vi "PPAS_DRIVE_EXECUTE.vi"(6 "Pass_Through_Time":dbl=-1.0 format="%33.4f", 8 "error in (no error)":errorcluster) -> (0 "error out":errorcluster)   [LabVIEW 2019]
uses:
  <vilib>/Rock Robotics/WPI/ThirdParty/JAS_Junk/TrajLib/Trajectory_Library.lvlib
  PPAS_DRIVE_GLOBALS.vi
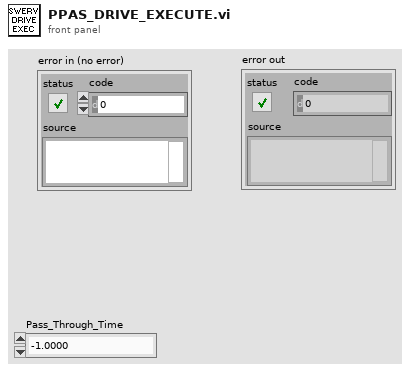
[diagram p1: front panel]
types:
  T1 = typedef "PPAS_DRIVE_MODULE_TYPDEF.ctl" = cluster{"SwervDriveMotor":T2, "SwerveSwerveMotor":T2, "SwerveDriveEnc":T7, "SwerveSwerveEnc":T7}
  T2 = typedef "WPI_MotorControlDeviceRef.ctl" = cluster{"DeviceStatus":errorcluster, "Type":T3, "PWM":cluster{"PWM Channel":T4, "DeadBand":T5}, "CAN":cluster{"Device Number":u8, "SetOutput VI Ref":variant, "GetOutput VI Ref":variant, "Enable VI Ref":variant, "Disable VI Ref":variant, "Data":variant}, "Invert":bool, "DIO PWM":cluster{"PWM \"Enable\" Channel":T4, "DIOChannel":T6, "PWM Rate":dbl}}
  T3 = typedef "WPI_MotorControlType.ctl" = enum16{"PWM", "CAN", "DIO PWM"}
  T4 = typedef "FPGA_DIOPWMChannel.ctl" = enum8{"PWM 0", "PWM 1", "PWM 2", "PWM 3", "PWM 4", "PWM 5", "PWM 6", "PWM 7", "PWM 8", "PWM 9", "PWM MXP 0", "PWM MXP 1", "PWM MXP 2", "PWM MXP 3", "PWM MXP 4", "PWM MXP 5", "PWM MXP 6", "PWM MXP 7", "PWM MXP 8", "PWM MXP 9", "Invalid"}
  T5 = typedef "WPI_PWMDeadband.ctl" = cluster{"Name":string, "maxPositivePwm":i32, "minPositivePwm":i32, "centerPwm":i32, "maxNegativePwm":i32, "minNegativePwm":i32, "angularRange":u16}
  T6 = typedef "FPGA_DIOChannel.ctl" = enum8{"DIO 0", "DIO 1", "DIO 2", "DIO 3", "DIO 4", "DIO 5", "DIO 6", "DIO 7", "DIO 8", "DIO 9", "DIO MXP 0", "DIO MXP 1", "DIO MXP 2", "DIO MXP 3", "DIO MXP 4", "DIO MXP 5", "DIO MXP 6", "DIO MXP 7", "DIO MXP 8", "DIO MXP 9", "DIO MXP 10", "DIO MXP 11", "DIO MXP 12", "DIO MXP 13", "DIO MXP 14", "DIO MXP 15", "SPI Port CS1", "SPI Port CS2", "SPI Port CS3", "SPI Port MISO", "SPI Port MOSI", "Invalid"}
  T7 = typedef "WPI_EncoderDevRef.ctl" = cluster{"DevStatus":errorcluster, "EncoderIndex":T8, "CounterIndex":T9, "DistancePerCount":dbl, "Decoding Type":T10}
  T8 = typedef "FPGA_EncoderIdx.ctl" = enum8{"Enc 0", "Enc 1", "Enc 2", "Enc 3", "Enc 4", "Enc 5", "Enc 6", "Enc 7", "Invalid"}
  T9 = typedef "FPGA_CounterCtrSystemIndex.ctl" = enum8{"Ctr 0", "Ctr 1", "Ctr 2", "Ctr 3", "Ctr 4", "Ctr 5", "Ctr 6", "Ctr 7", "Invalid"}
  T10 = typedef "WPI_EncoderType.ctl" = enum16{"1x", "2x", "4x"}
  T11 = typedef "WPI_GyroDevRef.ctl" = cluster{"DevStatus":errorcluster, "Analog Channel":T12, "Gain (VoltsPerDegree/Second)":dbl, "Gyro Type":enum16{"Analog", "XRS450"}, "Handle":i32, "SPI Bus":T13, "Device Found":bool, "Sample Rate":dbl, "Calibrate On Open":bool, "Offset":dbl}
  T12 = typedef "FPGA_AIChannel.ctl" = enum8{"AI 0", "AI 1", "AI 2", "AI 3", "AI MXP 0", "AI MXP 1", "AI MXP 2", "AI MXP 3", "Invalid"}
  T13 = typedef "spi_bus.ctl" = enum16{"SPI On-Board, CS0", "SPI On-Board, CS1", "SPI On-Board, CS2", "SPI On-Board, CS3", "SPI MXP", "Invalid"}
  T14 = typedef "Trajectory_Library.lvlib/SWERVE_DRIVE_MODULE_STATE.ctl" = cluster{"Speed":dbl, "Angle":T15}
  T15 = typedef "Trajectory_Library.lvlib/ROTATION2D.ctl" = cluster{"VALUE":dbl, "COS":dbl, "SIN":dbl}
  T16 = typedef "Trajectory_Library.lvlib/SWERVE_DRIVE_MODULE_POSITION.ctl" = cluster{"Distance":dbl, "Angle":T15, "P":bool}
  T17 = typedef "Trajectory_Library.lvlib/SWERVE_DRIVE_KINEMATICS.ctl" = cluster{"NumModules":i32, "InverseKinematics":T18, "ForwardKinematics":T18, "Modules":T19[], "PrevCoR":T19, "SavedModuleStates":T14[]}
  T18 = typedef "NI_Matrix.lvlib/RealMatrix.ctl" = dbl[][]
  T19 = typedef "Trajectory_Library.lvlib/TRANSLATION2D.ctl" = cluster{"X":dbl, "Y":dbl}
  T20 = typedef "Trajectory_Library.lvlib/CHASSIS_SPEEDS.ctl" = cluster{"vX":dbl, "vY":dbl, "vOmega":dbl}
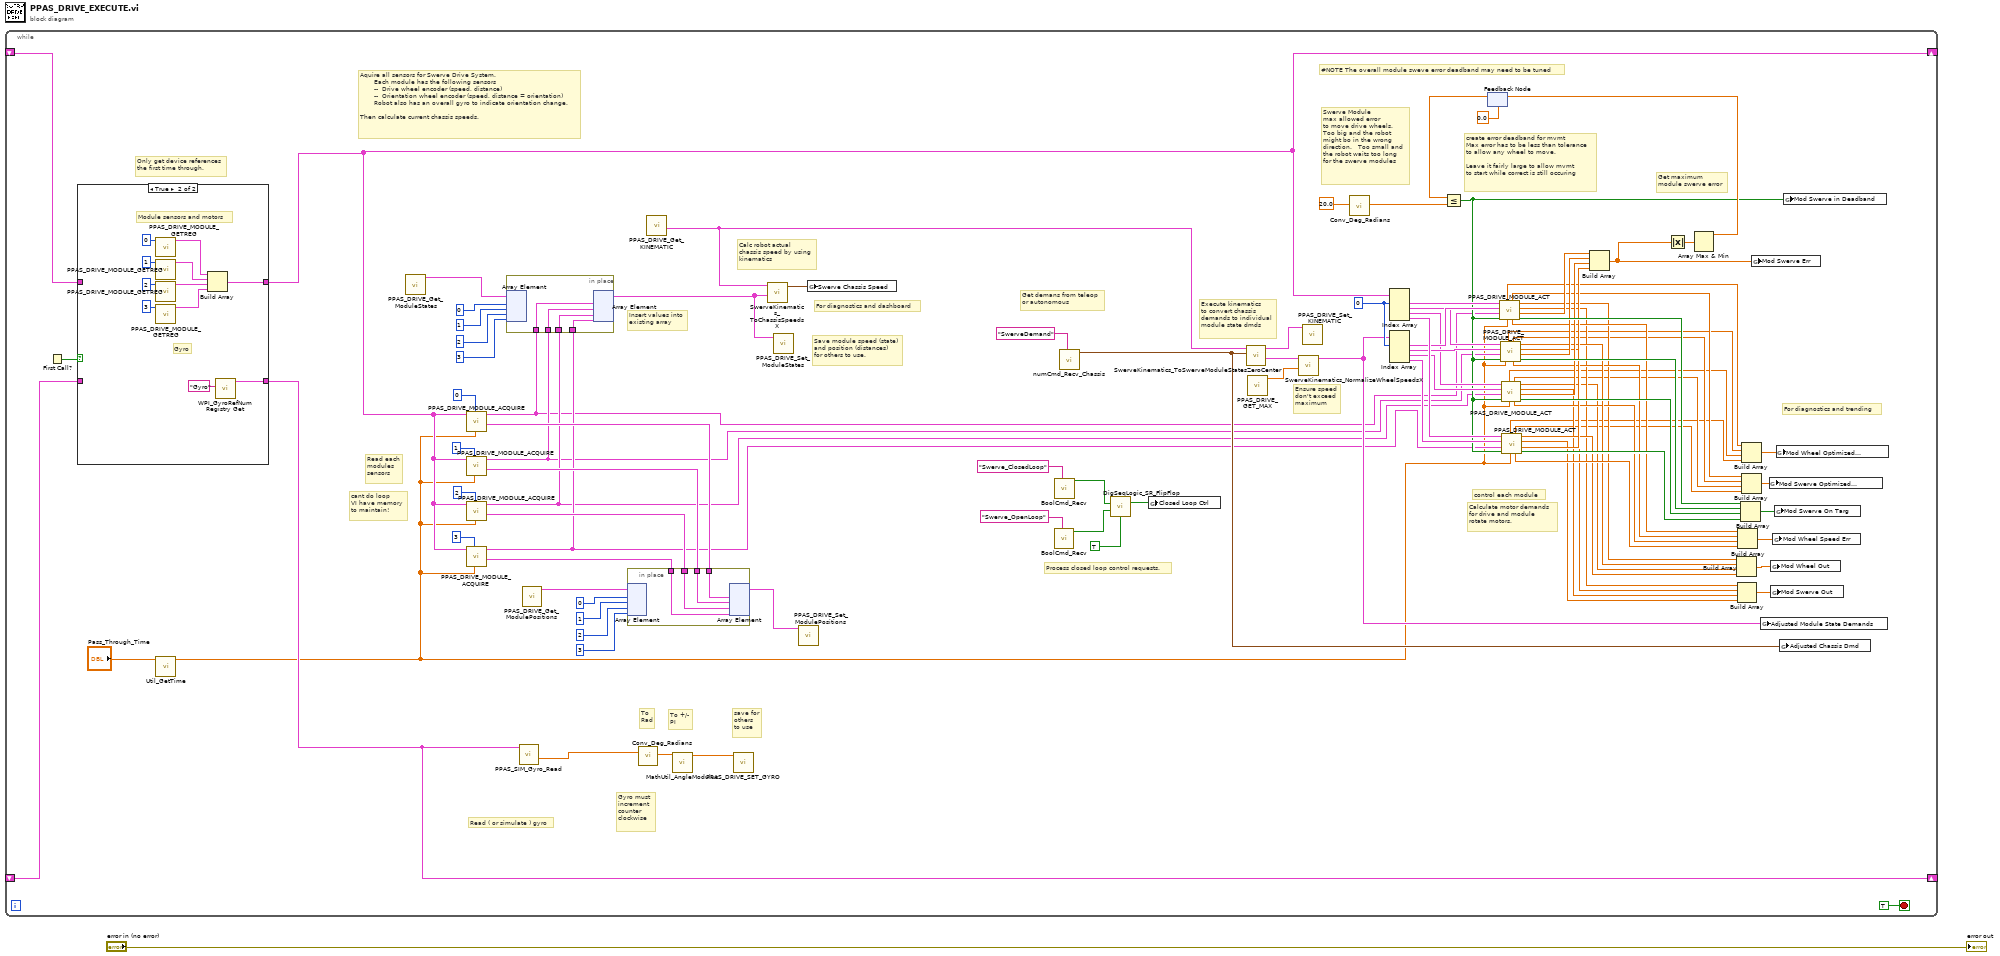
[diagram p0: block diagram]
diagram:
  n1 = while {
    shift-right: [w25] -> _
    shift-left: _ -> [w26]
    shift-right: [w24] -> _
    shift-left: _ -> [w23]
    stop <- TRUE stop-if-true
    w80 = 0 ("index")
    # "Process closed loop control requests."
    # "Only get device references\nthe first time through."
    # "save for\nothers\nto use"
    # "For diagnostics and trending"
    # "Insert values into\nexisting array"
    # "For diagnostics and dashboard"
    # "Read each\nmodules\nsensors"
    # "Gyro must\nincrement \ncounter\nclockwise"
    # "To +/-\nPI"
    # "To\nRad"
    # "Read ( or simulate ) gyro"
    # "Aquire all sensors for Swerve Drive System.\n       Each module has the following sensors\n       --  Drive wheel encoder (speed, distance)\n       --  Orientation wheel encoder (speed, distance = orientation)\n       Robot also has an overall gyro to indicate orientation change.\n\nThen calculate current chassis speeds."
    # "Calc robot actual\nchassis speed by using\nkinematics"
    # "Save module speed (state)\nand position (distances)\nfor others to use."
    # "cant do loop\nVI have memory\nto maintain!"
    # "Swerve Module\nmax allowed error\nto move drive wheels.\nToo big and the robot\nmight bo in the wrong\ndirection.   Too small and\nthe robot waits too long\nfor the swerve modules"
    # "Ensure speed\ndon't exceed\nmaximum"
    # "Get maximum \nmodule swerve error"
    # "#NOTE The overall module sweve error deadband may need to be tuned"
    # "create error deadband for mvmt\nMax error has to be less than tolerance\nto allow any wheel to move. \n\nLeave it fairly large to allow mvmt\nto start while correct is still occuring"
    # "Calculate motor demands\nfor drive and module \nrotate motors."
    # "Execute kinematics\nto convert chassis \ndemands to individual\nmodule state dmds"
    # "Get demans from teleop\nor autonomous"
    # "control each module"
    n2 = First Call?() -> (First Call?: T/F=w27:bool)
    n3 = case shown="True" w27 {
      tunnel: [w103 w110] -> w25
      tunnel: [w102 w109] -> w24
      tunnel: w26 -> [w103 _]
      tunnel: w23 -> [w102 _]
      frame False {
      }
      frame True {
        # "Module sensors and motors"
        # "Gyro"
        n4 = call "PPAS_DRIVE_MODULE_GETREG.vi"("Suffix"=0) -> ("Swerve Module TypDef"=w111:T1)  [unwired: 10 in]
        n5 = call "PPAS_DRIVE_MODULE_GETREG.vi"("Suffix"=1) -> ("Swerve Module TypDef"=w112:T1)  [unwired: 10 in]
        n6 = call "PPAS_DRIVE_MODULE_GETREG.vi"("Suffix"=2) -> ("Swerve Module TypDef"=w113:T1)  [unwired: 10 in]
        n7 = call "PPAS_DRIVE_MODULE_GETREG.vi"("Suffix"=3) -> ("Swerve Module TypDef"=w114:T1)  [unwired: 10 in]
        n8 = Build Array(w111, w112, w113, w114) -> (w110:T1[])
        n9 = call <vilib>:"WPI_GyroRefNum Registry Get.vi"("refnum name"="Gyro") -> ("GyroDevRef"=w109:T11)  [unwired: 9 in, 1 out]
      }
    }
    n10 = call <vilib>:"Util_GetTime.vi"("Pass_Through_Time"="Pass_Through_Time") -> ("FPGA_Time_Seconds"=w18:dbl)  [unwired: 8 in, 2 out]
    n11 = call "PPAS_DRIVE_Get_ModuleStates.vi"() -> ("Swerve Module States"=w33:T14[])  [unwired: 11 in]
    n12 = call "PPAS_DRIVE_MODULE_ACQUIRE.vi"("Pass_Through_Time"=w18, "Swerve Module Inx"=1, "Swerve Module TypDef"=w25) -> ("SWERVE DRIVE MODULE POSITION"=w43:T16, "Swerve Module State"=w20:T14)  [unwired: 7 in]
    n13 = call "PPAS_DRIVE_MODULE_ACQUIRE.vi"("Pass_Through_Time"=w18, "Swerve Module Inx"=3, "Swerve Module TypDef"=w25) -> ("SWERVE DRIVE MODULE POSITION"=w41:T16, "Swerve Module State"=w22:T14)  [unwired: 7 in]
    n14 = call "PPAS_DRIVE_MODULE_ACQUIRE.vi"("Pass_Through_Time"=w18, "Swerve Module Inx"=0, "Swerve Module TypDef"=w25) -> ("SWERVE DRIVE MODULE POSITION"=w44:T16, "Swerve Module State"=w8:T14)  [unwired: 7 in]
    n15 = call "PPAS_DRIVE_MODULE_ACQUIRE.vi"("Pass_Through_Time"=w18, "Swerve Module Inx"=2, "Swerve Module TypDef"=w25) -> ("SWERVE DRIVE MODULE POSITION"=w42:T16, "Swerve Module State"=w21:T14)  [unwired: 7 in]
    n16 = in-place {
      in-place-border: w8 -> [w118]
      in-place-border: w20 -> [w117]
      in-place-border: w21 -> [w116]
      in-place-border: w22 -> [w115]
      n17 = in-place-array #1(w33, 0, 1, 2, 3) -> ()  [unwired: 4 out]
      n18 = in-place-array #1(w118, w117, w116, w115) -> (w30:T14[])  [unwired: 4 out]
    }
    n19 = call "PPAS_SIM_Gyro_Read.vi"("GyroDevRef"=w24) -> ("Gyro_Cont_Deg"=w36:dbl)  [unwired: 10 in]
    n20 = call "PPAS_DRIVE_Get_ModulePositions.vi"() -> ("Swerve Module Positions"=w32:T16[])  [unwired: 11 in]
    n21 = in-place {
      in-place-border: w44 -> [w122]
      in-place-border: w43 -> [w121]
      in-place-border: w42 -> [w120]
      in-place-border: w41 -> [w119]
      n22 = in-place-array #2(w32, 0, 1, 2, 3) -> ()  [unwired: 4 out]
      n23 = in-place-array #2(w122, w121, w120, w119) -> (w31:T16[])  [unwired: 4 out]
    }
    n24 = call <vilib>:"Conv_Deg_Radians.vi"("Degress"=w36) -> ("Radians"=w54:dbl)  [unwired: 10 in]
    n25 = call "PPAS_DRIVE_Get_KINEMATIC.vi"() -> ("out SWERVE_DRIVE_KINEMATICS"=w35:T17)  [unwired: 11 in]
    n26 = call <vilib>:"MathUtil_AngleModulus.vi"("InputAngle"=w54) -> ("ModulsAngle"=w29:dbl)  [unwired: 10 in]
    n27 = call "PPAS_DRIVE_SET_GYRO.vi"("Gyro Heading Radians"=w29) -> ()  [unwired: 11 in]
    n28 = call <vilib>:"SwerveKinematics_ToChassisSpeedsX.vi"("WheelStates"=w30, "in SWERVE_DRIVE_KINEMATICS"=w35) -> ("Chassis Speed"=w53:T20)  [unwired: 9 in]
    n29 = call "PPAS_DRIVE_Set_ModuleStates.vi"("Swerve Module States"=w30) -> ()  [unwired: 11 in]
    n30 = call "PPAS_DRIVE_Set_ModulePositions.vi"("Swerve Module Positions"=w31) -> ()  [unwired: 11 in]
    n31 = global write "PPAS_DRIVE_GLOBALS.vi" "Swerve Chassis Speed"(w53) -> ()
    n32 = call <vilib>:"BoolCmd_Recv.vi"("Command Name"="Swerve_OpenLoop") -> ("New Request"=w4:bool)  [unwired: 9 in, 1 out]
    n33 = call <vilib>:"BoolCmd_Recv.vi"("Command Name"="Swerve_ClosedLoop") -> ("New Request"=w5:bool)  [unwired: 9 in, 1 out]
    n34 = call <vilib>:"numCmd_Recv_Chassis.vi"("Command Name"="SwerveDemand") -> ("Chassis Speeds"=w34:T20)  [unwired: 8 in, 2 out]
    n35 = call <vilib>:"DigSeqLogic_SR_FlipFlop.vi"("Set"=w5, "Reset"=w4, "Initial Value"=TRUE) -> ("Output"=w2:bool)  [unwired: 11 in, 1 out]
    n36 = global write "PPAS_DRIVE_GLOBALS.vi" "Closed Loop Ctrl"(w2) -> ()
    n37 = call <vilib>:"SwerveKinematics_ToSwerveModuleStatesZeroCenter.vi"("ChassisSpeeds"=w34, "in SWERVE_DRIVE_KINEMATICS"=w35) -> ("ModuleStates"=w67:T14[], "out SWERVE_DRIVE_KINEMATICS"=w57:T17)  [unwired: 8 in]
    n38 = call "PPAS_DRIVE_GET_MAX.vi"() -> ("Max Wheel Vel (Meter/Sec)"=w68:dbl)  [unwired: 10 in, 1 out]
    n39 = call <vilib>:"SwerveKinematics_NormalizeWheelSpeedsX.vi"("AttainableMaxSpeed"=w68, "in WheelStates"=w67) -> ("out WheelStates"=w59:T14[])  [unwired: 9 in]
    n40 = call "PPAS_DRIVE_Set_KINEMATIC.vi"("SWERVE_DRIVE_KINEMATICS"=w57) -> ()  [unwired: 11 in]
    n41 = call <vilib>:"Conv_Deg_Radians.vi"("Degress"=20.0 ("x")) -> ("Radians"=w56:dbl)  [unwired: 10 in]
    n42 = Index Array(array=w59, index #1=w80) -> (element #1=w72:T14, element #2=w73:T14, element #3=w74:T14, element #4=w84:T14)  [unwired: 3 in]
    n43 = Index Array(array=w25, index #1=w80) -> (element #1=w69:T1, element #2=w70:T1, element #3=w71:T1, element #4=w83:T1)  [unwired: 3 in]
    n44 = feedback #3(0.0) -> (w101:dbl)
    n45 = Less Or Equal?(x=w101, y=w56) -> (x <= y?=w62:bool)
    n46 = call "PPAS_DRIVE_MODULE_ACT.vi"("Pass_Through_Time"=w18, "AllSwervePosInDeadband"=w62, "Swerve State"=w8, "Swerve Dmd"=w72, "Swerve Module TypDef"=w69) -> ("SwerveOnTarget"=w94:bool, "SwervePosError"=w89:dbl, "Swerve Motor Dmd"=w77:dbl, "Wheel Motor Dmd"=w75:dbl, "WheelSpeedErr"=w85:dbl, "Optimized Swerve \nDmd Radians"=w19:dbl, "Optimized Speed \nDmd M/S"=w13:dbl)
    n47 = call "PPAS_DRIVE_MODULE_ACT.vi"("Pass_Through_Time"=w18, "AllSwervePosInDeadband"=w62, "Swerve State"=w20, "Swerve Dmd"=w73, "Swerve Module TypDef"=w70) -> ("SwerveOnTarget"=w95:bool, "SwervePosError"=w90:dbl, "Swerve Motor Dmd"=w78:dbl, "Wheel Motor Dmd"=w88:dbl, "WheelSpeedErr"=w86:dbl, "Optimized Swerve \nDmd Radians"=w17:dbl, "Optimized Speed \nDmd M/S"=w12:dbl)
    n48 = call "PPAS_DRIVE_MODULE_ACT.vi"("Pass_Through_Time"=w18, "AllSwervePosInDeadband"=w62, "Swerve State"=w21, "Swerve Dmd"=w74, "Swerve Module TypDef"=w71) -> ("SwerveOnTarget"=w96:bool, "SwervePosError"=w91:dbl, "Swerve Motor Dmd"=w79:dbl, "Wheel Motor Dmd"=w76:dbl, "WheelSpeedErr"=w87:dbl, "Optimized Swerve \nDmd Radians"=w16:dbl, "Optimized Speed \nDmd M/S"=w11:dbl)
    n49 = call "PPAS_DRIVE_MODULE_ACT.vi"("Pass_Through_Time"=w18, "AllSwervePosInDeadband"=w62, "Swerve State"=w22, "Swerve Dmd"=w84, "Swerve Module TypDef"=w83) -> ("SwerveOnTarget"=w97:bool, "SwervePosError"=w92:dbl, "Swerve Motor Dmd"=w82:dbl, "Wheel Motor Dmd"=w81:dbl, "WheelSpeedErr"=w93:dbl, "Optimized Swerve \nDmd Radians"=w15:dbl, "Optimized Speed \nDmd M/S"=w10:dbl)
    n50 = Build Array(w89, w90, w91, w92) -> (w64:dbl[])
    n51 = Absolute Value(x=w64) -> (abs(x)=w98:dbl[])
    n52 = Array Max & Min(array=w98) -> (max value=w99:dbl)  [unwired: 3 out]
    n53 = feedback-in #3(w99) -> ()
    n54 = Build Array(w75, w88, w76, w81) -> (w66:dbl[])
    n55 = Build Array(w77, w78, w79, w82) -> (w65:dbl[])
    n56 = Build Array(w85, w86, w87, w93) -> (w63:dbl[])
    n57 = Build Array(w94, w95, w96, w97) -> (w61:bool[])
    n58 = Build Array(w13, w12, w11, w10) -> (w9:dbl[])
    n59 = Build Array(w19, w17, w16, w15) -> (w14:dbl[])
    n60 = global write "PPAS_DRIVE_GLOBALS.vi" "Mod Swerve Err"(w64) -> ()
    n61 = global write "PPAS_DRIVE_GLOBALS.vi" "Adjusted Module State Demands"(w59) -> ()
    n62 = global write "PPAS_DRIVE_GLOBALS.vi" "Mod Swerve Optimized\nDmd"(w14) -> ()
    n63 = global write "PPAS_DRIVE_GLOBALS.vi" "Mod Wheel Out"(w66) -> ()
    n64 = global write "PPAS_DRIVE_GLOBALS.vi" "Mod Swerve Out"(w65) -> ()
    n65 = global write "PPAS_DRIVE_GLOBALS.vi" "Mod Wheel Speed Err"(w63) -> ()
    n66 = global write "PPAS_DRIVE_GLOBALS.vi" "Mod Swerve On Targ"(w61) -> ()
    n67 = global write "PPAS_DRIVE_GLOBALS.vi" "Mod Wheel Optimized \nDmd"(w9) -> ()
    n68 = global write "PPAS_DRIVE_GLOBALS.vi" "Adjusted Chassis Dmd"(w34) -> ()
    n69 = global write "PPAS_DRIVE_GLOBALS.vi" "Mod Swerve in Deadband"(w62) -> ()
  }
  "error out" <- "error in (no error)"
